vi "Validate Channel Name.vi"(8 "error in":errorcluster, 10 "channel name":string, 11 "routing channels in":T1 format="%.0x") -> (0 "error out":errorcluster, 3 "routing channels out":T1 format="%.0x")   [LabVIEW 2020, in "Routing and Faulting Scripting.lvlib"]
uses:
  Routing and Faulting Scripting.lvlib
  <vilib>/NI VeriStand/Custom Device API/Custom Device Item Ref.ctl
  <vilib>/NI VeriStand/Custom Device API/Custom Device API.lvlib
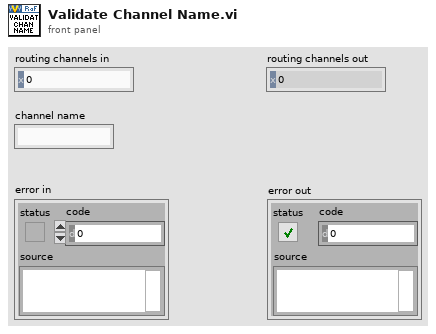
[diagram p1: front panel]
types:
  T1 = typedef "Custom Device API.lvlib/Custom Device Item Ref.ctl" = u64
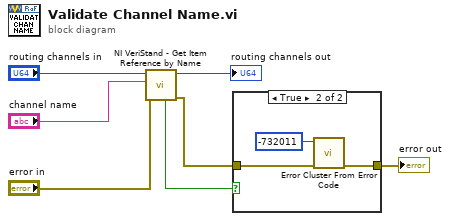
[diagram p0: block diagram]
diagram:
  n1 = call <vilib>:"NI VeriStand - Get Item Reference by Name.vi"("error in (no error)"="error in", "Item Name"="channel name", "Parent Ref in"="routing channels in") -> ("error out"=w3:errorcluster, "Parent Ref out"=→"routing channels out":T1, "Found"=w4:bool)  [unwired: 5 in, 1 out]
  n2 = case shown="True" w4 {
    tunnel: w3 -> [w8 w10]
    tunnel: [w8 w9] -> w2
    frame False {
    }
    frame True {
      n3 = call <vilib>:"Error Cluster From Error Code.vi"("error in (no error)"=w10, "error code (0)"=-732011) -> ("error out"=w9:errorcluster)  [unwired: 7 in]
    }
  }
  "error out" <- w2
